vi "GDSIconEditor_FileNameFilter_Dialog.vi"(8 "error in":errorcluster) -> (0 "error out":errorcluster, 2 "Cancelled":bool, 3 "FileNameConverions":T1)   [LabVIEW 2020]
uses:
  GDSIconEditor_FileNameFilter.ctl
panel:
  in  "Cancel":bool
  in  "Continue":bool
  in  "ClearConvertList":bool
  in  "ClearRemoveList":bool
  in  "Strings To Convert From - To":cluster{"From":string, "To":string}[](array[cluster])
  in  "String/Match Pattern to remove":string[](array[string])
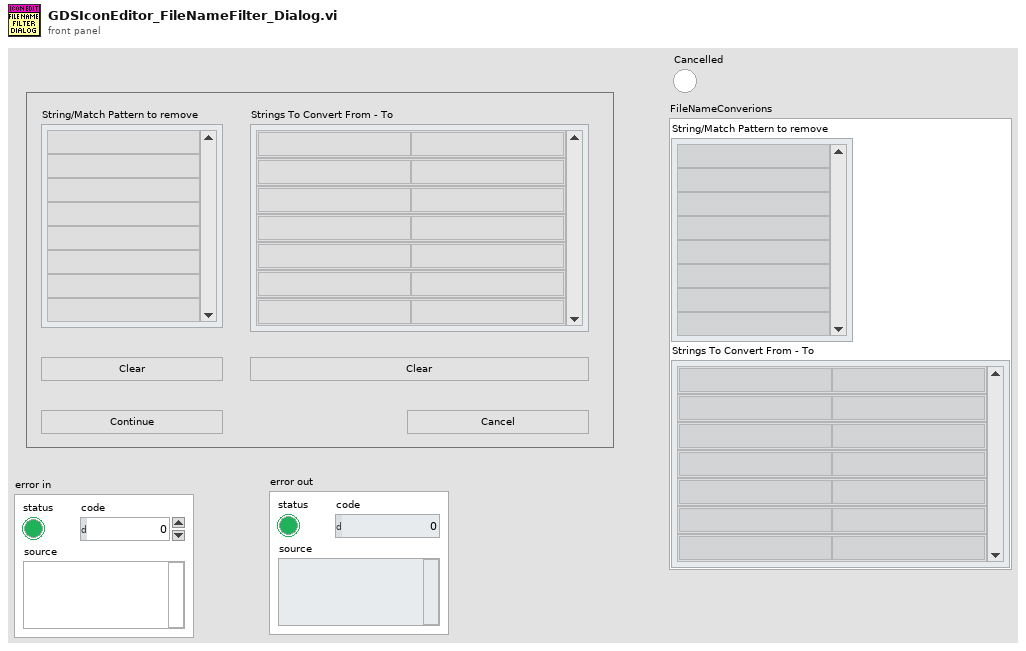
[diagram p1: front panel]
types:
  T1 = typedef "GDSIconEditor_FileNameFilter.ctl" = cluster{"String/Match Pattern to remove":string[], "Strings To Convert From - To":cluster{"From":string, "To":string}[]}
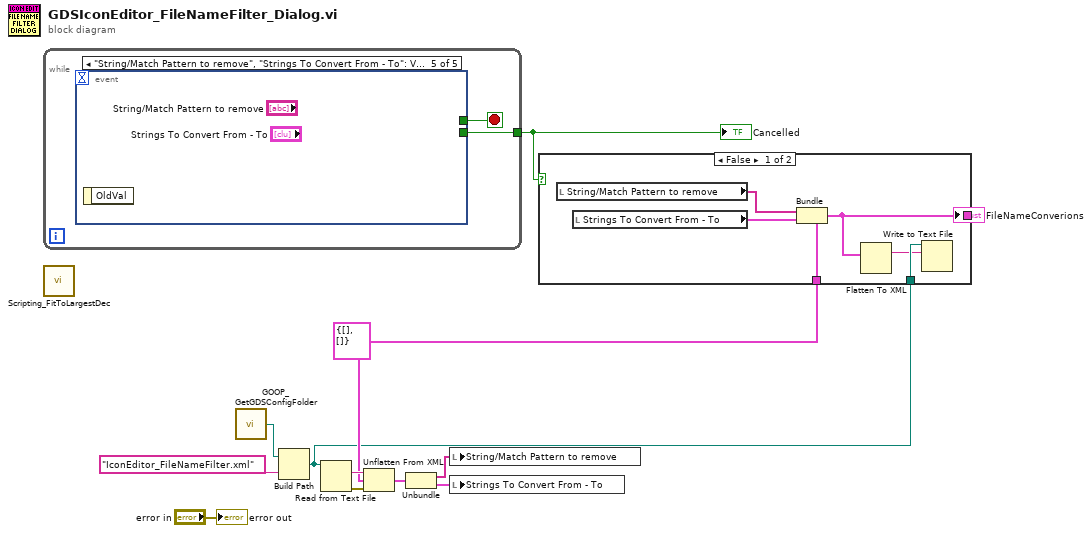
[diagram p0: block diagram]
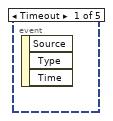
[diagram p3: hidden frame]
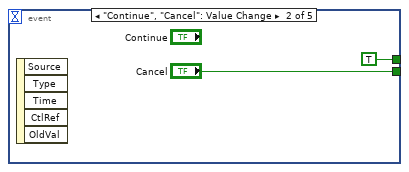
[diagram p4: hidden frame]
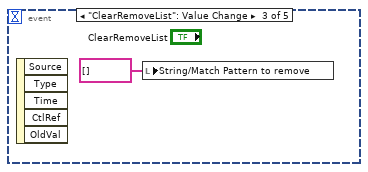
[diagram p5: hidden frame]
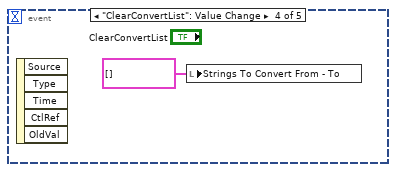
[diagram p6: hidden frame]
diagram:
  w2 = T1 {"String/Match Pattern to remove"=[], "Strings To Convert From - To"=[]} ("FileNameConverions")
  n1 = while {
    tunnel: [w13] -> w12
    stop <- w14 stop-if-true
    n2 = event shown="[4] \"String/Match Pattern to remove\", \"Strings To Convert From - To\": Value Change" {
      selector: _ -> [_ _ _ _ _]
      dyn-events: _ -> [_ _ _ _ _]
      timeout: _ -> [_ _ _ _ _]
      tunnel: [_ TRUE _ _ _] -> w14
      tunnel: [_ "Cancel" _ _ _] -> w13
      event Timeout {
        n3 = event-data() -> ()  [unwired: 1 in, 3 out]
      }
      event "Continue", "Cancel": Value Change {
        n4 = event-data() -> ()  [unwired: 1 in, 5 out]
      }
      event "ClearRemoveList": Value Change {
        n5 = event-data() -> ()  [unwired: 1 in, 5 out]
        n6 = local write "String/Match Pattern to remove"(string[] [] ("String/Match Pattern to remove")) -> ()
      }
      event "ClearConvertList": Value Change {
        n7 = event-data() -> ()  [unwired: 1 in, 5 out]
        n8 = local write "Strings To Convert From - To"(cluster{"From":string, "To":string}[] [] ("Strings To Convert From - To")) -> ()
      }
      event "String/Match Pattern to remove", "Strings To Convert From - To": Value Change {
        n9 = event-data() -> ()  [unwired: 1 in, 1 out]
      }
    }
  }
  "Cancelled" <- w12
  n10 = call "Scripting_FitToLargestDec.vi"() -> ()  [unwired: 6 in, 2 out]
  n11 = call "GOOP_GetGDSConfigFolder.vi"() -> ("GDSFolderPath"=w11:path)
  n12 = Build Path(base path=w11, name or relative path="IconEditor_FileNameFilter.xml") -> (appended path=w1:path)
  n13 = Read from Text File(file (use dialog)=w1) -> (text=w8:string, error out=w9:errorcluster)  [unwired: 3 in, 2 out]
  n14 = Unflatten From XML(xml string=w8, type=w2, error in (no error)=w9) -> (value=w7:T1)  [unwired: 1 out]
  n15 = Unbundle(w7) -> ("String/Match Pattern to remove"=w6:string[], "Strings To Convert From - To"=w5:cluster{"From":string, "To":string}[])
  n16 = local write "String/Match Pattern to remove"(w6) -> ()
  n17 = local write "Strings To Convert From - To"(w5) -> ()
  n18 = case shown="False" w12 {
    tunnel: [w21 _] -> w3
    tunnel: w2 -> [w22 _]
    tunnel: w1 -> [w20 _]
    frame False {
      n19 = local read "String/Match Pattern to remove"() -> (w24:string[])
      n20 = local read "Strings To Convert From - To"() -> (w23:cluster{"From":string, "To":string}[])
      n21 = Bundle(cluster=w22, "String/Match Pattern to remove"=w24, "Strings To Convert From - To"=w23) -> (w21:T1)
      n22 = Flatten To XML(6:w21) -> (2:w19:string)
      n23 = Write to Text File(file (use dialog)=w20, text=w19) -> ()  [unwired: 2 in, 3 out]
    }
    frame True {
    }
  }
  "FileNameConverions" <- w3
  "error out" <- "error in"
